vi "Load Macro from File.vi"(8 "error in (no error)":errorcluster, 11 "Path":path) -> (0 "error out":errorcluster, 3 "Macro":refnum<class "Macro.lvclass">)   [LabVIEW 2020, in "MacroAssert.lvlib"]
doc: "Loads a macro from <B>Path</B>."
uses:
  MacroAssert.lvlib
  Macro/Macro.lvclass
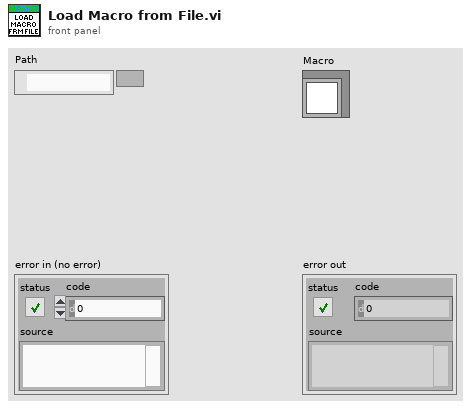
[diagram p1: front panel]
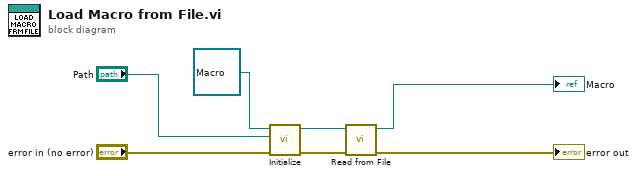
[diagram p0: block diagram]
diagram:
  n1 = call-dynamic "Initialize.vi"("error in (no error)"="error in (no error)", "Path"="Path", "Macro in"=refnum<class "Macro.lvclass"> refnum) -> ("error out"=w6:errorcluster, "Macro out"=w2:refnum<class "Macro.lvclass">)  [unwired: 7 in]
  n2 = call-dynamic "Read from File.vi"("error in (no error)"=w6, "Macro in"=w2) -> ("error out"=→"error out":errorcluster, "Macro out"=→"Macro":refnum<class "Macro.lvclass">)  [unwired: 8 in]
